vi "Count Paths.vi"(7 "constraints":string[](array[string]), 8 "error in (no error)":errorcluster, 9 "destination":string, 10 "source":string, 11 "Topological Sort in":refnum<class "Topological Sort.lvclass">) -> (0 "error out":errorcluster, 2 "Number of Paths":u64, 3 "Topological Sort out":refnum<class "Topological Sort.lvclass">)   [LabVIEW 2025, in "AOC.lvlib" / "Topological Sort.lvlib" / "Topological Sort.lvclass"]
uses:
  Topological Sort.lvclass
  Topological Sort.lvclass/Topological Sort.ctl
  <vilib>/Utility/miscctls.llb/LVMapReplaceAction.ctl
  Graph/Graph.lvclass
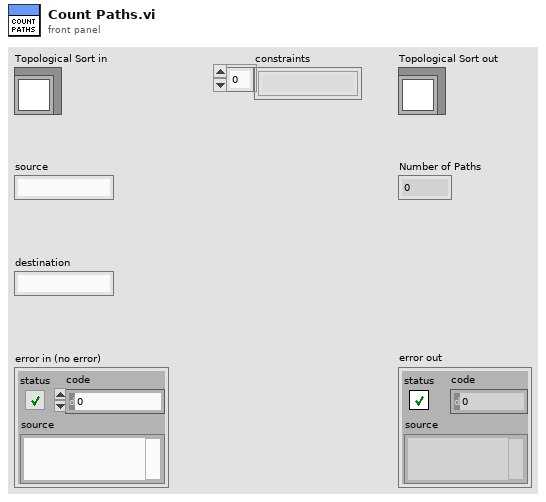
[diagram p1: front panel]
types:
  T1 = typedef "LVMapReplaceAction.ctl" = enum32{"Modify Entry only if found", "Add or Modify Entry", "Delete Entry"}
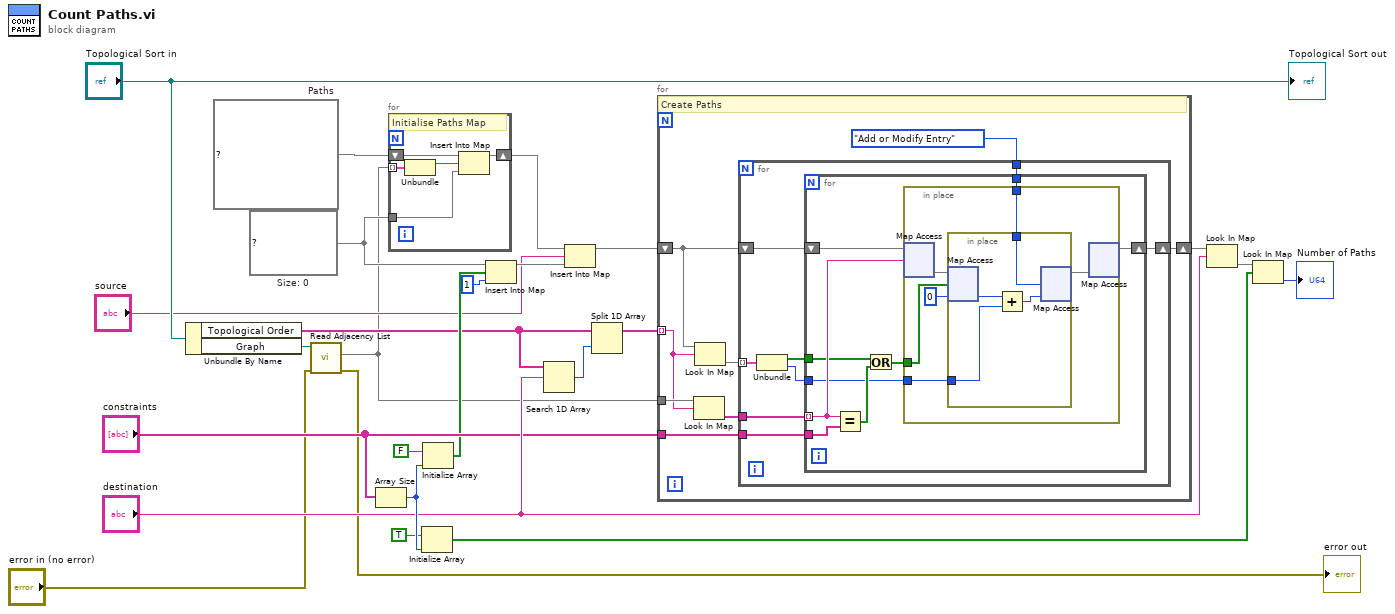
[diagram p0: block diagram]
diagram:
  w14 = map{bool[], u64} {}  # Size: 0
  w6 = map{string, map{bool[], u64}} {}  # Paths
  n1 = Unbundle By Name("Topological Sort in") -> ("Topological Order"=w5:string[], "Graph"=w4:refnum<class "Graph.lvclass">)
  n2 = call-dynamic "Read Adjacency List.vi"("error in (no error)"="error in (no error)", "Graph in"=w4) -> ("error out"=→"error out":errorcluster, "Adjacency List"=w2:map{string, string[]})  [unwired: 7 in, 1 out]
  n3 = Array Size(array="constraints") -> (size(s)=w22:i32)
  n4 = for {
    tunnel: w2 -> [w28] mode=indexing
    shift-right: [w29] -> w7
    shift-left: w6 -> [w30]
    tunnel: w14 -> [w27]
    # "Initialise Paths Map"
    n5 = Unbundle(w28) -> (w26:string)  [unwired: 1 out]
    n6 = Insert Into Map(map in=w30, key=w26, value=w27) -> (map out=w29:map{string, map{bool[], u64}})  [unwired: 2 out]
  }
  n7 = Initialize Array(TRUE, w22) -> (w24:bool[])
  n8 = Initialize Array(FALSE ("Boolean"), w22) -> (w15:bool[])
  n9 = Insert Into Map(map in=w14, key=w15, value=u64 1) -> (map out=w17:map{bool[], u64})  [unwired: 2 out]
  n10 = Search 1D Array(1D array=w5, element="destination") -> (index of element=w12:i32)  [unwired: 1 in]
  n11 = Insert Into Map(map in=w7, key="source", value=w17) -> (map out=w9:map{string, map{bool[], u64}})  [unwired: 2 out]
  n12 = Split 1D Array(array=w5, index=w12) -> (first subarray=w10:string[])  [unwired: 1 out]
  n13 = for {
    tunnel: w10 -> [w36] mode=indexing
    shift-right: [w33] -> w19
    shift-left: w9 -> [w34]
    tunnel: w2 -> [w37]
    tunnel: "constraints" -> [w32]
    # "Create Paths"
    n14 = Look In Map(map=w37, key=w36) -> (value=w35:string[])  [unwired: 1 in, 1 out]
    n15 = Look In Map(map=w34, key=w36) -> (value=w38:map{bool[], u64})  [unwired: 1 in, 1 out]
    n16 = for {
      tunnel: w38 -> [w45] mode=indexing
      tunnel: w35 -> [w46]
      shift-right: [w42] -> w33
      shift-left: w34 -> [w43]
      tunnel: w32 -> [w41]
      tunnel: LVMapReplaceAction."Add or Modify Entry" ("action") -> [w40]
      n17 = Unbundle(w45) -> (w44:bool[], w39:u64)
      n18 = for {
        tunnel: w46 -> [w52] mode=indexing
        tunnel: w44 -> [w51]
        shift-right: [w54] -> w42
        shift-left: w43 -> [w55]
        tunnel: w41 -> [w53]
        tunnel: w40 -> [w48]
        tunnel: w39 -> [w47]
        n19 = Equal?(x=w52, y=w53) -> (x = y?=w50:bool[])
        n20 = Or(x=w51, y=w50) -> (x .or. y?=w49:bool[])
        n21 = in-place {
          in-place-border: w49 -> [w60]
          in-place-border: w48 -> [w59]
          in-place-border: w47 -> [w57]
          n22 = in-place-map #1(w55, w52) -> (w61:map{bool[], u64})  [unwired: 1 in, 1 out]
          n23 = in-place {
            in-place-border: w59 -> [w65]
            in-place-border: w57 -> [w63]
            n24 = in-place-map #2(w61, w60, u64 0) -> (w64:u64)  [unwired: 1 out]
            n25 = Add(x=w64, y=w63) -> (x+y=w62:u64)
            n26 = in-place-map #2(w62, w65) -> (w56:map{bool[], u64})  [unwired: 2 out]
          }
          n27 = in-place-map #1(w56) -> (w54:map{string, map{bool[], u64}})  [unwired: 1 in, 2 out]
        }
      }
    }
  }
  n28 = Look In Map(map=w19, key="destination") -> (value=w23:map{bool[], u64})  [unwired: 1 in, 1 out]
  n29 = Look In Map(map=w23, key=w24) -> (value=→"Number of Paths":u64)  [unwired: 1 in, 1 out]
  "Topological Sort out" <- "Topological Sort in"
